vi "Read Background Image (SubVI).vi"(11 "File REF In":refnum<file>) -> (0 "BG Image":T1={"Ipl Header Size"=112, "ID"=0, "N Channels"=1, "Alpha Channel"=0, "Depth"=8, "Color Model"=1497453127, "Color Sequence"=1497453127, "Data Order"=0, "Origin"=0, "Align"=4, "Width"=1770, "Height"=1728, "ROI"=0, "Mask ROI"=0, "Image ID"=0, "Title Info"=0, "Image Size"=4091904, "Image Data"=1109131328, "Width Step"=2368, "Border Mode"=0, "Border Const"=0, "Image Data Origin"=0, "BG Image"=[]}, 3 "File REF Out":refnum<file>)   [LabVIEW 2015]
uses:
  Controls/BG Image.ctl
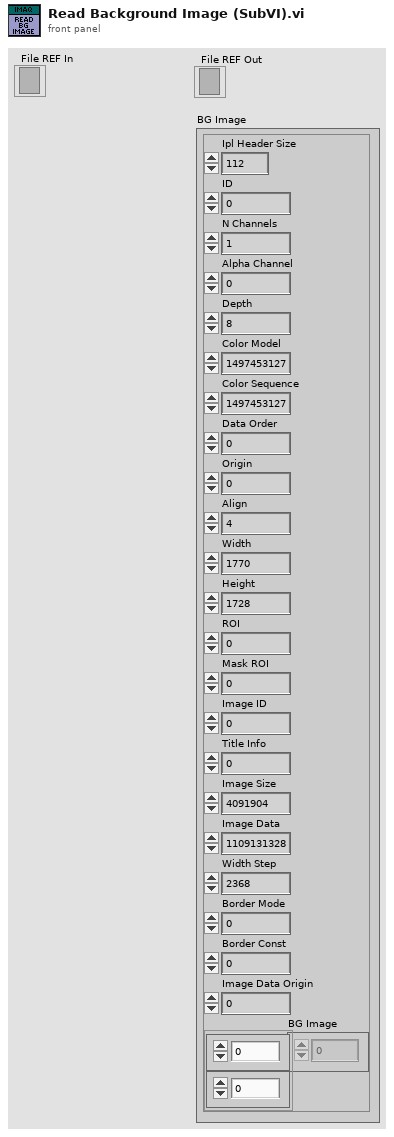
[diagram p1: front panel]
types:
  T1 = typedef "BG Image.ctl" = cluster{"Ipl Header Size":i32, "ID":i32, "N Channels":i32, "Alpha Channel":i32, "Depth":i32, "Color Model":i32, "Color Sequence":i32, "Data Order":i32, "Origin":i32, "Align":i32, "Width":i32, "Height":i32, "ROI":i32, "Mask ROI":i32, "Image ID":i32, "Title Info":i32, "Image Size":i32, "Image Data":i32, "Width Step":i32, "Border Mode":i32, "Border Const":i32, "Image Data Origin":i32, "BG Image":u8[][]}
  T2 = enum16{"big-endian, network order", "native, host order", "little-endian"}
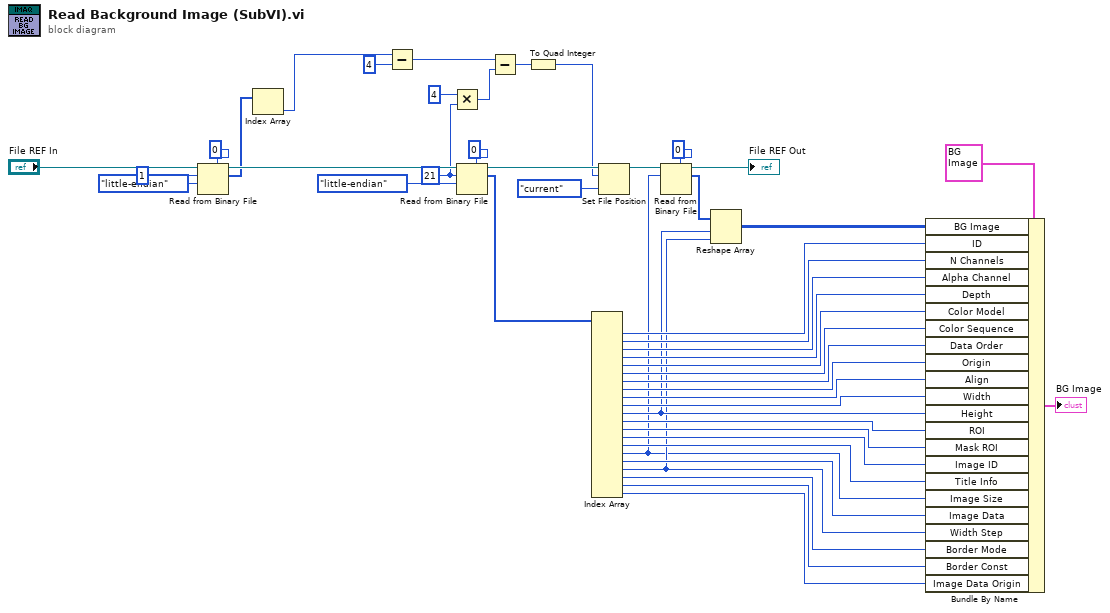
[diagram p0: block diagram]
diagram:
  w28 = 21 ("count (1)")
  n1 = Read from Binary File(5:0, 9:T2."little-endian" ("byte order (0:big-endian, network order)"), 10:1 ("count (1)"), 11:"File REF In") -> (2:w34:i32[], 3:w41:refnum<file>)  [unwired: 2 in, 2 out]
  n2 = Index Array(array=w34) -> (element=w30:i32)  [unwired: 1 in]
  n3 = Subtract(x=w30, y=4) -> (x-y=w26:i32)
  n4 = Multiply(x=4, y=w28) -> (x*y=w25:i32)
  n5 = Read from Binary File(5:0, 9:T2."little-endian" ("byte order (0:big-endian, network order)"), 10:w28, 11:w41) -> (2:w39:i32[], 3:w43:refnum<file>)  [unwired: 2 in, 2 out]
  n6 = Subtract(x=w26, y=w25) -> (x-y=w24:i32)
  n7 = To Quad Integer(1:w24) -> (0:w23:i64)
  n8 = Index Array(array=w39) -> (element #1=w31:i32, element #2=w20:i32, element #3=w19:i32, element #4=w18:i32, element #5=w17:i32, element #6=w16:i32, element #7=w15:i32, element #8=w14:i32, element #9=w13:i32, element #10=w12:i32, element #11=w11:i32, element #12=w10:i32, element #13=w9:i32, element #14=w8:i32, element #15=w7:i32, element #16=w1:i32, element #17=w6:i32, element #18=w5:i32, element #19=w4:i32, element #20=w3:i32, element #21=w2:i32)  [unwired: 21 in]
  n9 = Set File Position(offset (in bytes) (0)=w23, refnum=w43, from (0:start)=enum16{"start", "end", "current"}."current") -> (refnum out=w45:refnum<file>)  [unwired: 1 in, 1 out]
  n10 = Read from Binary File(5:u8 0, 10:w1, 11:w45) -> (2:w46:u8[], 3:→"File REF Out":refnum<file>)  [unwired: 3 in, 2 out]
  n11 = Reshape Array(w46, w11, w5) -> (w21:u8[][])
  n12 = Bundle By Name(cluster=T1 {"Ipl Header Size"=112, "ID"=0, "N Channels"=1, "Alpha Channel"=0, "Depth"=8, "Color Model"=1497453127, "Color Sequence"=1497453127, "Data Order"=0, "Origin"=0, "Align"=4, "Width"=1770, "Height"=1728, "ROI"=0, "Mask ROI"=0, "Image ID"=0, "Title Info"=0, "Image Size"=4091904, "Image Data"=1109131328, "Width Step"=2368, "Border Mode"=0, "Border Const"=0, "Image Data Origin"=0, "BG Image"=[]}, "BG Image"=w21, "ID"=w31, "N Channels"=w20, "Alpha Channel"=w19, "Depth"=w18, "Color Model"=w17, "Color Sequence"=w16, "Data Order"=w15, "Origin"=w14, "Align"=w13, "Width"=w12, "Height"=w11, "ROI"=w10, "Mask ROI"=w9, "Image ID"=w8, "Title Info"=w7, "Image Size"=w1, "Image Data"=w6, "Width Step"=w5, "Border Mode"=w4, "Border Const"=w3, "Image Data Origin"=w2) -> (→"BG Image":T1)
